vi "CRYASIOAddPlayBuffer.vi"(7 "Limit":i32=30000, 8 "Data Length":i32, 9 "pData":sgl[](array[numeric]), 10 "error in (no error)":errorcluster) -> (1 "Buffer Amount":i32, 2 "bResult":bool, 3 "error out":errorcluster)   [LabVIEW 2013]
uses:
  CRY_ASIO.dll
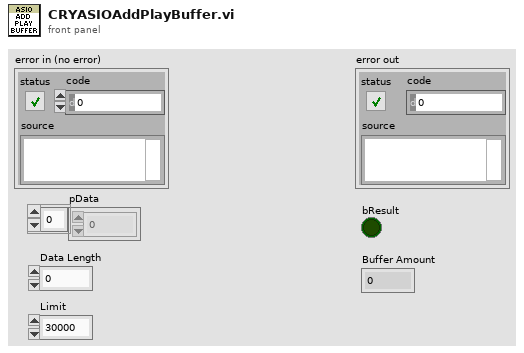
[diagram p1: front panel]
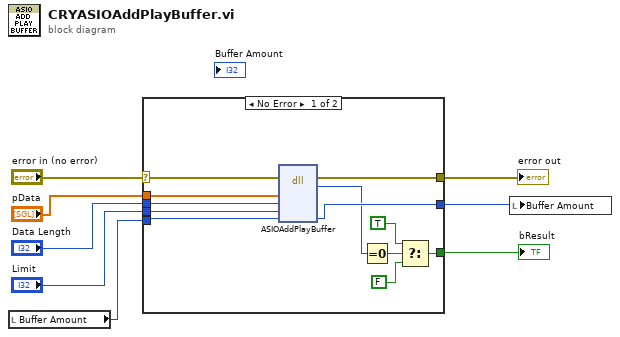
[diagram p0: block diagram]
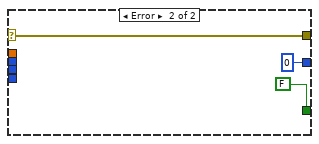
[diagram p2: hidden frame]
diagram:
  n1 = local read "Buffer Amount"() -> (w2:i32)
  n2 = case shown="No Error" "error in (no error)" {
    selector: "error in (no error)" -> [w16 w23]
    tunnel: [w15 w23] -> w7
    tunnel: [w17 FALSE] -> w6
    tunnel: "pData" -> [w14 _]
    tunnel: "Data Length" -> [w13 _]
    tunnel: "Limit" -> [w12 _]
    tunnel: w2 -> [w11 _]
    tunnel: [w10 0 ("arg4")] -> w1
    frame No Error {
      n3 = dll-call lib="D:/LabView_Project/CRY6181/CRY_ASIO.dll" fn="ASIOAddPlayBuffer"(error in=w16, "arg1"=w14, "arg2"=w13, "arg3"=w12, "arg4"=w11) -> (error out=w15:errorcluster, "return type"=w9:u32, "arg4"=w10:i32)  [unwired: 5 in, 1 out]
      n4 = Equal To 0?(x=w9) -> (x = 0?=w20:bool)
      n5 = Select(t=TRUE, s=w20, f=FALSE) -> (s? t:f=w17:bool)
    }
    frame Error {
    }
  }
  "error out" <- w7
  "bResult" <- w6
  n6 = local write "Buffer Amount"(w1) -> ()
